vi "HTTP_State.vi"(8 "error in (no error)":errorcluster) -> (0 "error out":errorcluster, 1 "Connected?":bool, 2 "GET Code":T1, 3 "Connection":string)   [LabVIEW 2020]
uses:
  RestAPI.ctl
  JSON_Formats.vi
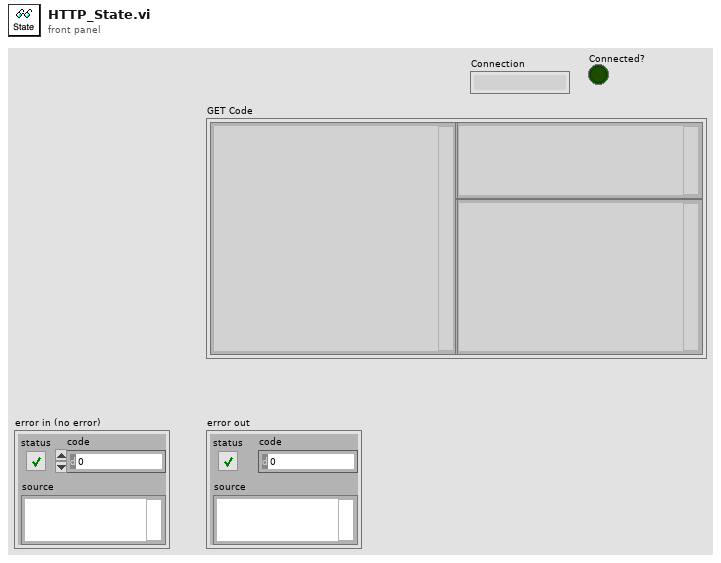
[diagram p1: front panel]
types:
  T1 = typedef "RestAPI.ctl" = cluster{"headers 2":string, "headers":string, "body":string}
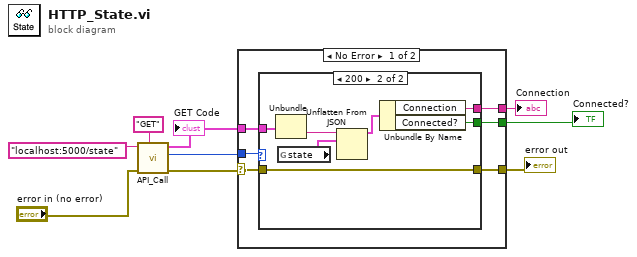
[diagram p0: block diagram]
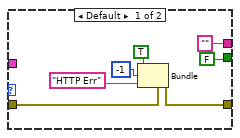
[diagram p2: hidden frame]
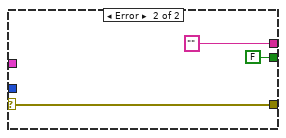
[diagram p3: hidden frame]
diagram:
  n1 = call "API_Call.vi"("Cmd"="GET" ("input 1"), "error in (no error)"="error in (no error)", "url"="localhost:5000/state") -> ("error out"=w6:errorcluster, "Err Code"=w5:i32, "Communication"=w8:T1)  [unwired: 6 in]
  "GET Code" <- w8
  n2 = case shown="No Error" w6 {
    selector: w6 -> [w14 w32]
    tunnel: w5 -> [w15 _]
    tunnel: [w13 w32] -> w7
    tunnel: w8 -> [w12 _]
    tunnel: [w11 "" ("REPL")] -> w9
    tunnel: [w10 FALSE ("Connected?")] -> w1
    frame No Error {
      n3 = case shown="200" w15 {
        tunnel: w14 -> [w22 w29]
        tunnel: [w21 w29] -> w13
        tunnel: w12 -> [_ w28]
        tunnel: ["" ("REPL") w25] -> w11
        tunnel: [FALSE ("Connected?") w24] -> w10
        frame Default {
          n4 = Bundle(cluster=w22, "status"=TRUE, "code"=-1, "source"="HTTP Err") -> (w21:errorcluster)
        }
        frame 200 {
          n5 = Unbundle(w28) -> ("body"=w27:string)  [unwired: 2 out]
          n6 = global read "JSON_Formats.vi" "state"() -> (w23:cluster{"Connection":string, "Connected?":bool})
          n7 = Unflatten From JSON(JSON string=w27, type and defaults=w23) -> (value=w26:cluster{"Connection":string, "Connected?":bool})  [unwired: 5 in, 1 out]
          n8 = Unbundle By Name(w26) -> ("Connection"=w25:string, "Connected?"=w24:bool)
        }
      }
    }
    frame Error {
    }
  }
  "Connection" <- w9
  "error out" <- w7
  "Connected?" <- w1
